vi "Get Message Sent Event.vi"(8 "Error In":errorcluster, 11 "reference in":refnum<class "Communicator.lvclass">) -> (0 "Error Out":errorcluster, 2 "Msg Sent Event":refnum<user-event>, 3 "reference out":refnum<class "Communicator.lvclass">)   [LabVIEW 2019, in "Communicator.lvclass"]
uses:
  Communicator.lvclass
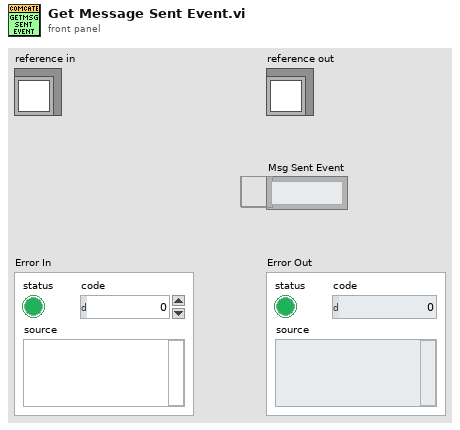
[diagram p1: front panel]
types:
  T1 = typedef "Communicator.lvclass/ObjectAttributes.ctl" = cluster{"IConfigure":refnum<class "IConfigure.lvclass">, "Worker Enqueuer":refnum<class "Message Enqueuer.lvclass">, "Start Counter":i32, "Msg Sent":refnum<user-event>}
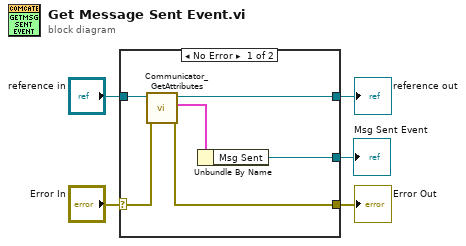
[diagram p0: block diagram]
diagram:
  n1 = case shown="No Error" "Error In" {
    selector: "Error In" -> [w11 w13]
    tunnel: [w9 w13] -> w4
    tunnel: [w7 w12] -> w2
    tunnel: "reference in" -> [w8 w12]
    tunnel: [w6 _] -> w1
    frame No Error {
      n2 = call "Communicator_GetAttributes.vi"("Error In"=w11, "Communicator in"=w8) -> ("Error Out"=w9:errorcluster, "Data"=w10:T1, "Communicator out"=w7:refnum<class "Communicator.lvclass">)  [unwired: 6 in, 1 out]
      n3 = Unbundle By Name(w10) -> ("Msg Sent"=w6:refnum<user-event>)
    }
    frame Error {
    }
  }
  "Error Out" <- w4
  "reference out" <- w2
  "Msg Sent Event" <- w1
